vi "Get Waveform Chart Plot Names.vi"(8 "error in (no error)":errorcluster, 11 "reference in":refnum<vi>) -> (0 "error out":errorcluster, 2 "Plot Names":string[](array[string]), 3 "reference out":refnum<vi>)   [LabVIEW 2018]
doc: "Gets the plot names in a waveform chart legend. Supports any waveform chart type."
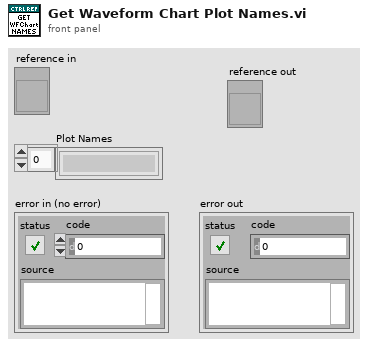
[diagram p1: front panel]
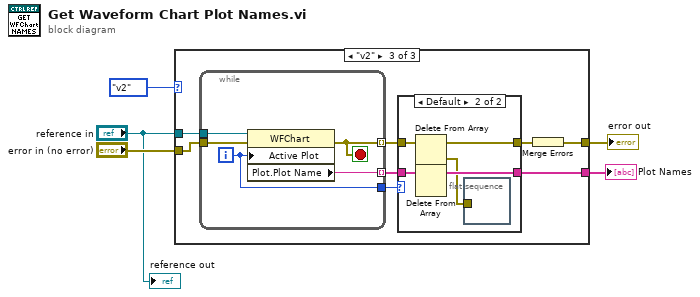
[diagram p0: block diagram]
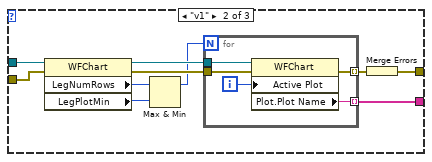
[diagram p3: hidden frame]
diagram:
  n1 = case shown="\"v2\"" enum16{"v1", "v2", "v3"}."v2" {
    tunnel: [w6 w16 w29] -> w5
    tunnel: "reference in" -> [_ w14 w28]
    tunnel: "error in (no error)" -> [w6 w13 w27]
    tunnel: [_ w12 w25] -> w3
    frame Default {
    }
    frame "v1" {
      n2 = property on="Property Node" class="WFChart"(reference=w14, error in=w13) -> (reference out=w10:refnum<vi>, error out=w11:errorcluster, "LegNumRows"=w9:u32, "LegPlotMin"=w8:u32)
      n3 = Max & Min(x=w9, y=w8) -> (max(x,y)=w7:u32)  [unwired: 1 out]
      n4 = for {
        N: w7 -> [_]
        tunnel: [w21] -> w15 mode=indexing
        tunnel: w10 -> [w20]
        tunnel: w11 -> [w19]
        tunnel: [w17] -> w12 mode=indexing
        i -> [w18]
        n5 = property on="Property Node" class="WFChart"(reference=w20, error in=w19, "Active Plot"=w18) -> (error out=w21:errorcluster, "Plot.Plot Name"=w17:string)  [unwired: 1 out]
      }
      n6 = Merge Errors(w15) -> (w16:errorcluster)
    }
    frame "v2" {
      n7 = while {
        tunnel: [w38] -> w24 mode=indexing
        tunnel: w28 -> [w41]
        tunnel: w27 -> [w40]
        tunnel: [w39] -> w26 mode=indexing
        tunnel: [w37] -> w22
        i -> [w37]
        stop <- w38 stop-if-true
        n8 = property on="Property Node" class="WFChart"(reference=w41, error in=w40, "Active Plot"=w37) -> (error out=w38:errorcluster, "Plot.Plot Name"=w39:string)  [unwired: 1 out]
      }
      n9 = case shown="Default" w22 {
        tunnel: w26 -> [w30 w36]
        tunnel: [w30 w35] -> w25
        tunnel: w24 -> [w31 w34]
        tunnel: [w31 w33] -> w23
        frame 1 {
        }
        frame Default {
          n10 = Delete From Array(array=w34) -> (deleted portion=w32:errorcluster, array with subset deleted=w33:errorcluster[])  [unwired: 2 in]
          n11 = Delete From Array(array=w36) -> (array with subset deleted=w35:string[])  [unwired: 2 in, 1 out]
          n12 = flat-sequence {
            tunnel: w32 -> [_]
            frame #0 {
            }
          }
        }
      }
      n13 = Merge Errors(w23) -> (w29:errorcluster)
    }
  }
  "Plot Names" <- w3
  "error out" <- w5
  "reference out" <- "reference in"
